vi "AG E3644A set.vi"() -> ()   [LabVIEW 2014]
panel:
  in  "current lim (A)":ext=1000.0 format="%.3f"
  in  "voltage (V)":ext=1000.0 format="%.3f"
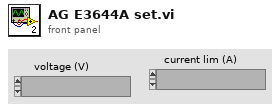
[diagram p1: front panel]
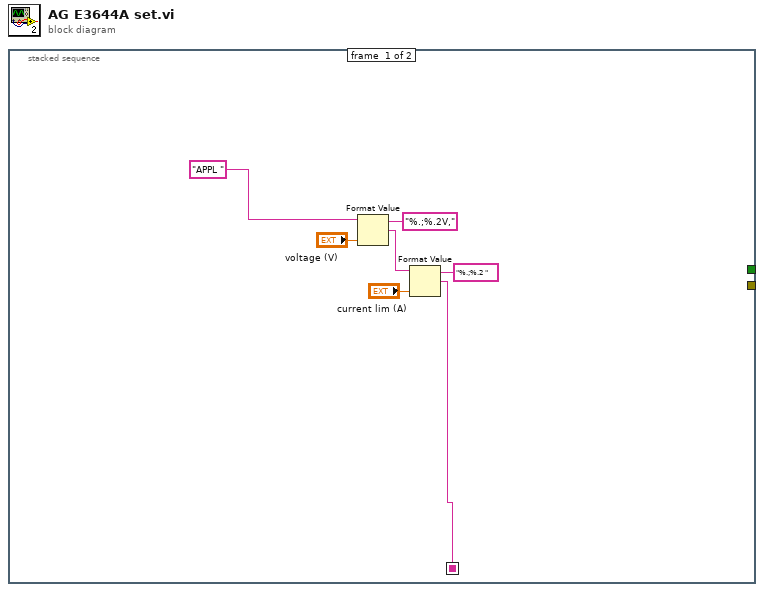
[diagram p0: block diagram]
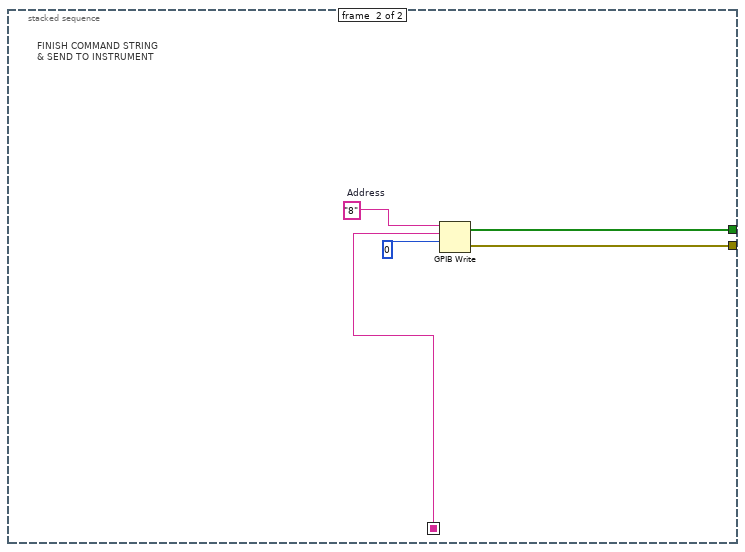
[diagram p2: hidden frame]
diagram:
  n1 = stacked-sequence {
    seq-local: [w1 _] -> [_ w8]
    tunnel: [_ w10] -> _
    tunnel: [_ w9] -> _
    frame #0 {
      n2 = Format Value(string ("")="APPL ", format string="%.;%.2V,", value (0)="voltage (V)") -> (output string=w2:string)
      n3 = Format Value(string ("")=w2, format string="%.;%.2 ", value (0)="current lim (A)") -> (output string=w1:string)
    }
    frame #1 {
      w11 = "8"  # Address
      # "FINISH COMMAND STRING\n& SEND TO INSTRUMENT"
      n4 = GPIB Write(0:w11, 1:w8, 2:0) -> (5:w10:bool[], 6:w9:errorcluster)  [unwired: 1 in, 1 out]
    }
  }
